vi "hex_to_dec.vi"(2 "begin from left side?":bool, 3 "Array":dbl[](array[numeric])) -> (1 "Numeric":dbl)   [LabVIEW 2023]
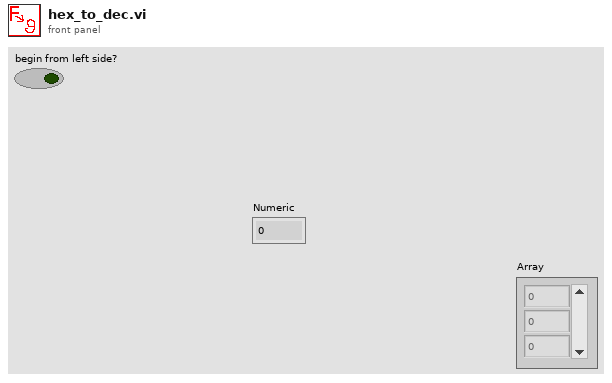
[diagram p1: front panel]
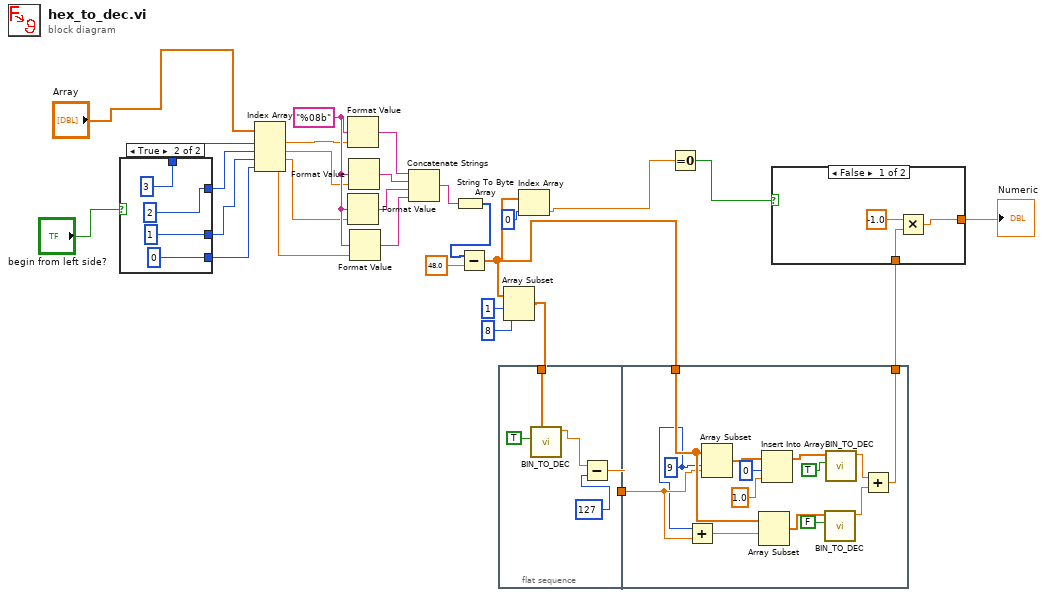
[diagram p0: block diagram]
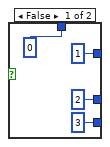
[diagram p2: hidden frame]
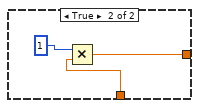
[diagram p3: hidden frame]
diagram:
  w15 = "%08b" ("format string")
  n1 = case shown="True" "begin from left side?" {
    tunnel: [1 ("index") 2 ("index")] -> w5
    tunnel: [0 ("index") 3 ("index")] -> w4
    tunnel: [2 ("index") 1 ("index")] -> w3
    tunnel: [3 ("index") 0 ("index")] -> w2
    frame False {
    }
    frame True {
    }
  }
  n2 = Index Array(array="Array", index #1=w4, index #2=w5, index #3=w3, index #4=w2) -> (element #1=w7:dbl, element #2=w12:dbl, element #3=w13:dbl, element #4=w14:dbl)
  n3 = Format Value(format string=w15, value (0)=w7) -> (output string=w8:string)  [unwired: 1 in]
  n4 = Format Value(format string=w15, value (0)=w13) -> (output string=w16:string)  [unwired: 1 in]
  n5 = Format Value(format string=w15, value (0)=w12) -> (output string=w9:string)  [unwired: 1 in]
  n6 = Format Value(format string=w15, value (0)=w14) -> (output string=w23:string)  [unwired: 1 in]
  n7 = Concatenate Strings(w8, w9, w16, w23) -> (w10:string)
  n8 = String To Byte Array(string=w10) -> (unsigned byte array=w22:u8[])
  n9 = Subtract(x=w22, y=48.0) -> (x-y=w25:dbl[])
  n10 = flat-sequence {
    tunnel: w24 -> [w39]
    tunnel: [w38] -> w28
    tunnel: w28 -> [w50]
    tunnel: w25 -> [w51]
    tunnel: [w42] -> w26
    frame #0 {
      n11 = call "BIN_TO_DEC.vi"("Before point?"=TRUE ("before point"), "Array"=w39) -> ("output"=w41:dbl)  [unwired: 9 in]
      n12 = Subtract(x=w41, y=127) -> (x-y=w38:dbl)
    }
    frame #1 {
      w49 = 9 ("index")
      n13 = Add(x=w49, y=w50) -> (x+y=w48:dbl)
      n14 = Array Subset(array=w51, index=w49, length=w50) -> (w54:dbl[])
      n15 = Array Subset(array=w51, index=w48) -> (w47:dbl[])  [unwired: 1 in]
      n16 = Insert Into Array(array=w54, index=0, new element=1.0 ("new element/subarray")) -> (w52:dbl[])
      n17 = call "BIN_TO_DEC.vi"("Before point?"=FALSE ("before point"), "Array"=w47) -> ("output"=w43:dbl)  [unwired: 9 in]
      n18 = call "BIN_TO_DEC.vi"("Before point?"=TRUE ("before point"), "Array"=w52) -> ("output"=w44:dbl)  [unwired: 9 in]
      n19 = Add(x=w44, y=w43) -> (x+y=w42:dbl)
    }
  }
  n20 = Array Subset(array=w25, index=1, length=8) -> (w24:dbl[])
  n21 = Index Array(array=w25, index=0) -> (element=w20:dbl)
  n22 = Equal To 0?(x=w20) -> (x = 0?=w17:bool)
  n23 = case shown="False" w17 {
    tunnel: w26 -> [w58 w60]
    tunnel: [w56 w59] -> w27
    frame False {
      n24 = Multiply(x=-1.0, y=w58) -> (x*y=w56:dbl)
    }
    frame True {
      n25 = Multiply(x=1, y=w60) -> (x*y=w59:dbl)
    }
  }
  "Numeric" <- w27
